vi "Index String.vi"(10 "N":i32, 11 "String":string) -> (3 "Indexed Strings":string[](array[string]))   [LabVIEW 2015, in "Teaching File.lvlib"]
doc: "Append N index decimal postfixes to the input string."
uses:
  Teaching File.lvlib
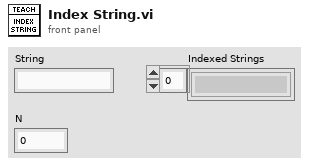
[diagram p1: front panel]
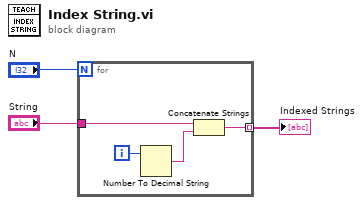
[diagram p0: block diagram]
diagram:
  n1 = for {
    N: "N" -> [_]
    tunnel: "String" -> [w5]
    tunnel: [w4] -> w3 mode=indexing
    i -> [w7]
    n2 = Number To Decimal String(number=w7) -> (decimal integer string=w6:string)  [unwired: 1 in]
    n3 = Concatenate Strings(w5, w6) -> (w4:string)
  }
  "Indexed Strings" <- w3
